vi "GV gated frameclock.vi"() -> ()   [LabVIEW 2017]
panel:
  out "Gated frameclock":bool
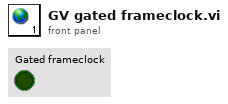
[diagram p1: front panel]
diagram:
